vi "00_EventStructure.vi"() -> ()   [LabVIEW 2019]
uses:
  <vilib>/Utility/miscctls.llb/LVPoint32TypeDef.ctl
panel:
  out "PlatMods 2":T1
  out "Mods 2":cluster{"Menu Key":bool}
  out "ButtonMods":T2
  out "Orientation":enum16{"Horizontal", "Vertical"}(ring)
  out "Delta":i32
  out "Time":u32
  out "CtlRef":refnum<vi>
  out "Coords":T3
  out "PlatMods":T1
  out "Mods":cluster{"Double Click":bool, "Menu Key":bool}
  out "Button 2":u16
  in  "Stop":bool
  out "Numeric":i32
  in  "Button":bool
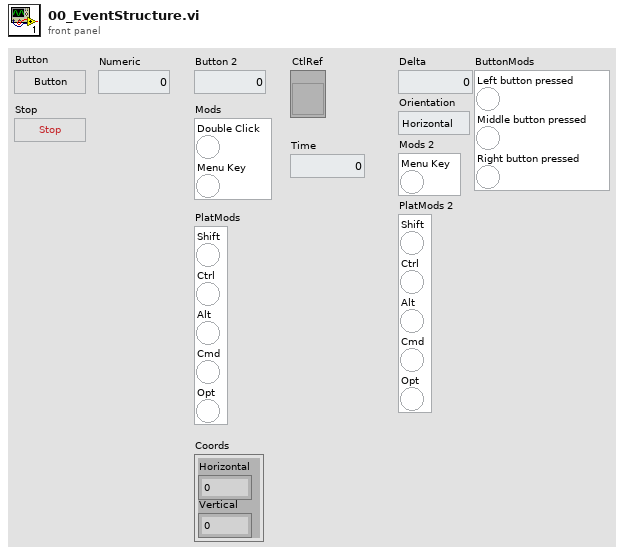
[diagram p1: front panel]
types:
  T1 = cluster{"Shift":bool, "Ctrl":bool, "Alt":bool, "Cmd":bool, "Opt":bool}
  T2 = cluster{"Left button pressed":bool, "Middle button pressed":bool, "Right button pressed":bool}
  T3 = typedef "LVPoint32TypeDef.ctl" = cluster{"Horizontal":i32, "Vertical":i32}
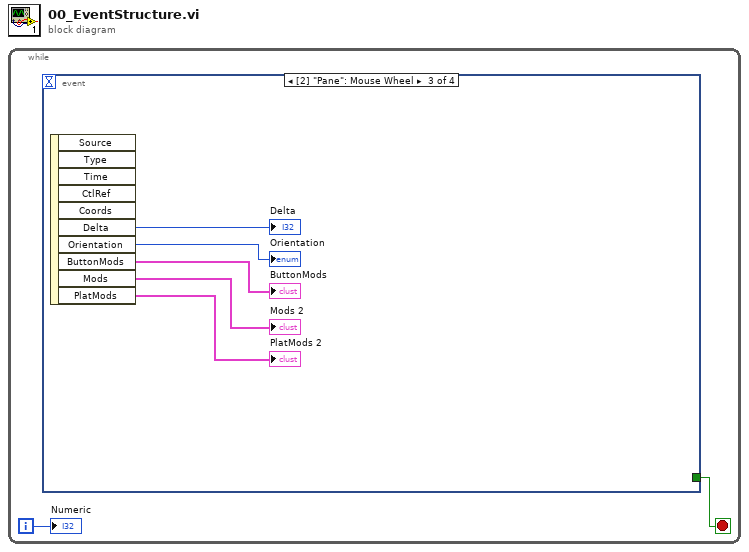
[diagram p0: block diagram]
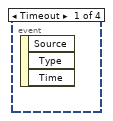
[diagram p2: hidden frame]
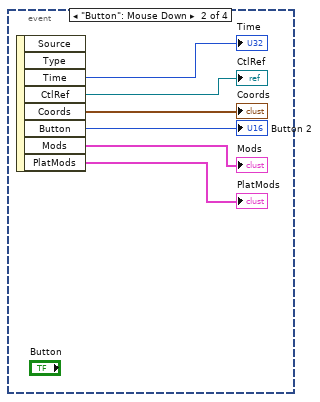
[diagram p3: hidden frame]
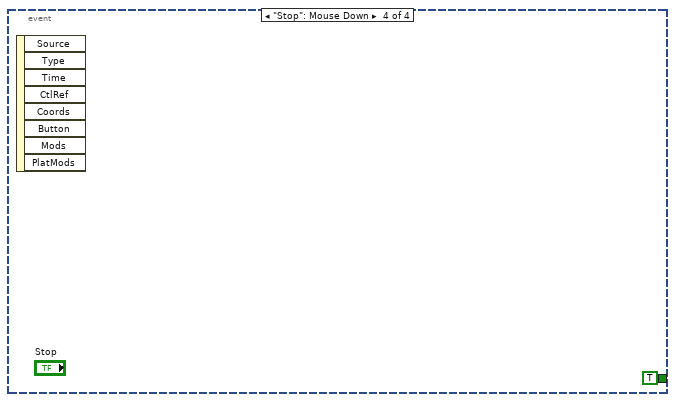
[diagram p4: hidden frame]
diagram:
  n1 = while {
    i -> [w2]
    stop <- w1 stop-if-true
    n2 = event shown="[2] \"Pane\": Mouse Wheel" {
      selector: _ -> [_ _ _ _]
      dyn-events: _ -> [_ _ _ _]
      timeout: _ -> [_ _ _ _]
      tunnel: [_ _ _ TRUE] -> w1
      event Timeout {
        n3 = event-data() -> ()  [unwired: 1 in, 3 out]
      }
      event "Button": Mouse Down {
        n4 = event-data() -> ("Time"=→"Time":u32, "CtlRef"=→"CtlRef":refnum<vi>, "Coords"=→"Coords":T3, "Button"=→"Button 2":u16, "Mods"=→"Mods":cluster{"Double Click":bool, "Menu Key":bool}, "PlatMods"=→"PlatMods":T1)  [unwired: 1 in, 2 out]
      }
      event Mouse Wheel {
        n5 = event-data() -> ("Delta"=→"Delta":i32, "Orientation"=→"Orientation":enum16{"Horizontal", "Vertical"}, "ButtonMods"=→"ButtonMods":T2, "Mods"=→"Mods 2":cluster{"Menu Key":bool}, "PlatMods"=→"PlatMods 2":T1)  [unwired: 1 in, 5 out]
      }
      event "Stop": Mouse Down {
        n6 = event-data() -> ()  [unwired: 1 in, 8 out]
      }
    }
    "Numeric" <- w2
  }
